vi "Run_Enter_Temp.vi"(1 "Wait until done":bool) -> (0 "error out":errorcluster)   [LabVIEW 2010]
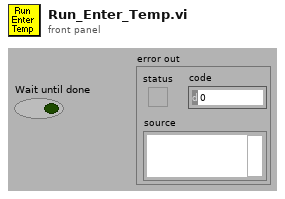
[diagram p1: front panel]
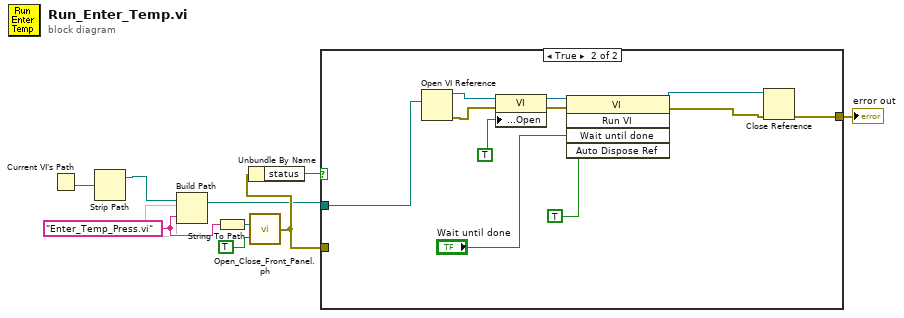
[diagram p0: block diagram]
diagram:
  w6 = "Enter_Temp_Press.vi" ("name or relative path")
  n1 = Current VI's Path() -> (path=w3:path)
  n2 = Strip Path(path=w3) -> (stripped path=w2:path)  [unwired: 1 out]
  n3 = Build Path(base path=w2, name or relative path=w6) -> (appended path=w8:path)
  n4 = String To Path(string=w6) -> (path=w5:path)
  n5 = call "Open_Close_Front_Panel.ph.vi"("Front Panel Window:Open"=TRUE, "VI path"=w5) -> ("error out"=w9:errorcluster)  [unwired: 1 out]
  n6 = Unbundle By Name(w9) -> ("status"=w7:bool)
  n7 = case shown="True" w7 {
    tunnel: w8 -> [_ w21]
    tunnel: [w10 w20] -> w1
    tunnel: w9 -> [w10 _]
    frame False {
    }
    frame True {
      n8 = Open VI Reference(vi path=w21) -> (vi reference=w18:refnum<vi>, error out=w17:errorcluster)  [unwired: 1 in, 4 out]
      n9 = property class="VI"(reference=w18, error in=w17, "Front Panel Window:Open"=TRUE) -> (reference out=w16:refnum<vi>, error out=w15:errorcluster)
      n10 = invoke class="VI" method="Run VI"(reference=w16, error in=w15, "Wait until done"="Wait until done", "Auto Dispose Ref"=TRUE) -> (reference out=w14:refnum<vi>, error out=w13:errorcluster)  [unwired: 1 in, 3 out]
      n11 = Close Reference(reference=w14, error in (no error)=w13) -> (error out=w20:errorcluster)
    }
  }
  "error out" <- w1
